vi "sub_table_laden.vi"(1 "Zeile":dbl, 2 "ItemNames":string[][](array[string])) -> (0 "Array":dbl[](array[numeric]))   [LabVIEW 2009]
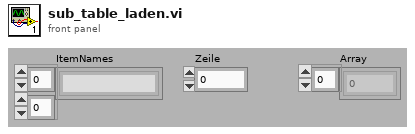
[diagram p1: front panel]
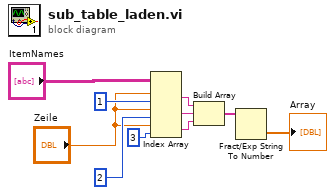
[diagram p0: block diagram]
diagram:
  n1 = Index Array(array="ItemNames", index (row) #1="Zeile", index (col) #1=1 ("Deaktivierter Index (Spalte)"), index (row) #2="Zeile", index (col) #2=2 ("Deaktivierter Index (Spalte)"), index (row) #3="Zeile", index (col) #3=3 ("Deaktivierter Index (Spalte)")) -> (element #1=w5:string, element #2=w6:string, element #3=w7:string)
  n2 = Build Array(w5, w6, w7) -> (w9:string[])
  n3 = Fract/Exp String To Number(string=w9) -> (number=→"Array":dbl[])  [unwired: 3 in, 1 out]
